vi "Write File Path.vi"(8 "error in (no error)":errorcluster, 10 "File Path":string, 11 "Setup File in":refnum<class "Setup File.lvclass">) -> (0 "error out":errorcluster, 3 "Setup File out":refnum<class "Setup File.lvclass">)   [LabVIEW 2018, in "Setup File.lvclass"]
doc: "Este VI escreve o caminho do arquivo na classe. Possui um código que acrescenta o caracter '\\\" ao final da string caso ele não exista."
uses:
  Setup File.lvclass
  Setup File.lvclass/Setup File.ctl
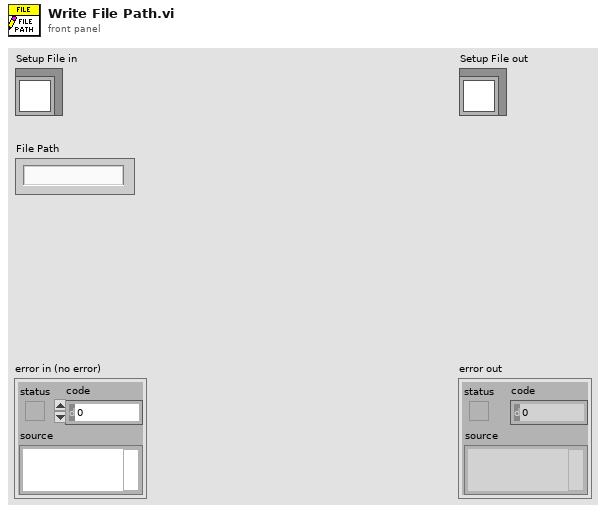
[diagram p1: front panel]
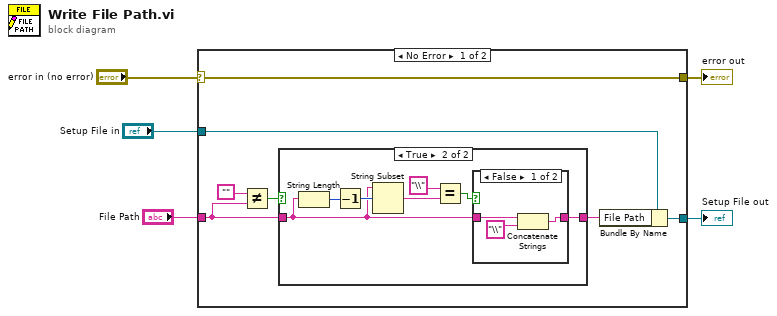
[diagram p0: block diagram]
diagram:
  n1 = case shown="No Error" "error in (no error)" {
    selector: "error in (no error)" -> [w12 w25]
    tunnel: [w12 w25] -> w4
    tunnel: [w10 w26] -> w2
    tunnel: "Setup File in" -> [w11 w26]
    tunnel: "File Path" -> [w7 _]
    frame No Error {
      n2 = Not Equal?(x="", y=w7) -> (x != y?=w8:bool)
      n3 = case shown="True" w8 {
        tunnel: w7 -> [w13 w15]
        tunnel: [w13 w14] -> w6
        frame False {
        }
        frame True {
          n4 = String Length(string=w15) -> (length=w20:i32)
          n5 = Decrement(x=w20) -> (x-1=w19:i32)
          n6 = String Subset(string=w15, offset (0)=w19) -> (substring=w18:string)  [unwired: 1 in]
          n7 = Equal?(x="\\", y=w18) -> (x = y?=w16:bool)
          n8 = case shown="False" w16 {
            tunnel: w15 -> [w23 w24]
            tunnel: [w21 w24] -> w14
            frame False {
              n9 = Concatenate Strings(w23, "\\" ("x")) -> (w21:string)
            }
            frame True {
            }
          }
        }
      }
      n10 = Bundle By Name(cluster=w11, "File Path"=w6) -> (w10:refnum<class "Setup File.lvclass">)
    }
    frame Error {
    }
  }
  "error out" <- w4
  "Setup File out" <- w2
